vi "Generate Simulated Data.vi"(8 "error in (no error)":T5 caption="entrée d'erreur (pas d'erreur)", 11 "Type de signal":T3) -> (0 "error out":T5 caption="sortie d'erreur", 2 "Données du graphe":waveform(dbl)[](array[waveform]))   [LabVIEW 2018, in "Acquisition.lvlib"]
doc: "Génère des exemples de waveforms en fonction du type de signal dans l'entrée Configuration du matériel."
uses:
  Acquisition.lvlib
  <vilib>/Analysis/NI_AALBase.lvlib
  Signal Type.ctl
  Hardware Configuration.ctl
  Logging/Logging Configuration.ctl
  Logging/Logging.lvlib
  Settings/Settings.ctl
  Settings/Settings.lvlib
panel:
  in  "Paramètres en entrée":T1={"Configuration du matériel"={"Refnum de matériel <À remplacer>"="", "Type de signal <À remplacer>"=enum."Sine Wave"}, "Configuration de l'enregistrement"={"Chemin de base du fichier journal"=path "", "Référence de fichier TDMS"=refnum}, "Mode de longueur d'onde"={"Choix du mode"=TRUE, "Commande numérique"=0.0}, "périphérique"={"Nom du périphérique"="Dev1"}}
  in  "S5":bool[](array[boolean])=[FALSE, TRUE, FALSE, TRUE]
  in  "S4":bool[](array[boolean])=[FALSE, TRUE, FALSE, FALSE]
  in  "S6":bool[](array[boolean])=[FALSE, TRUE, TRUE, FALSE]
  in  "S7":bool[](array[boolean])=[FALSE, TRUE, TRUE, TRUE]
  in  "S13":bool[](array[boolean])=[TRUE, TRUE, FALSE, TRUE]
  in  "S12":bool[](array[boolean])=[TRUE, TRUE, FALSE, FALSE]
  in  "S11":bool[](array[boolean])=[TRUE, FALSE, TRUE, TRUE]
  in  "S10":bool[](array[boolean])=[TRUE, FALSE, TRUE, FALSE]
  in  "S9":bool[](array[boolean])=[TRUE, FALSE, FALSE, TRUE]
  in  "S8":bool[](array[boolean])=[TRUE, FALSE, FALSE, FALSE]
  in  "S3":bool[](array[boolean])=[TRUE, TRUE, FALSE, FALSE]
  in  "S2":bool[](array[boolean])=[FALSE, TRUE, FALSE, FALSE]
  in  "S1":bool[](array[boolean])=[TRUE, FALSE, FALSE, FALSE]
  in  "S0":bool[](array[boolean])=[FALSE, FALSE, FALSE, FALSE]
  in  "nom du périphérique":tag="Dev1"
  out "Graphe déroulant":dynamicdata(graph)
  # "ALLO MON GROS TAPON\n\nCOMPTE TES SWITCH A L'ENDROIT AVANT QUE JE TE CASSE TES KNEECAP"
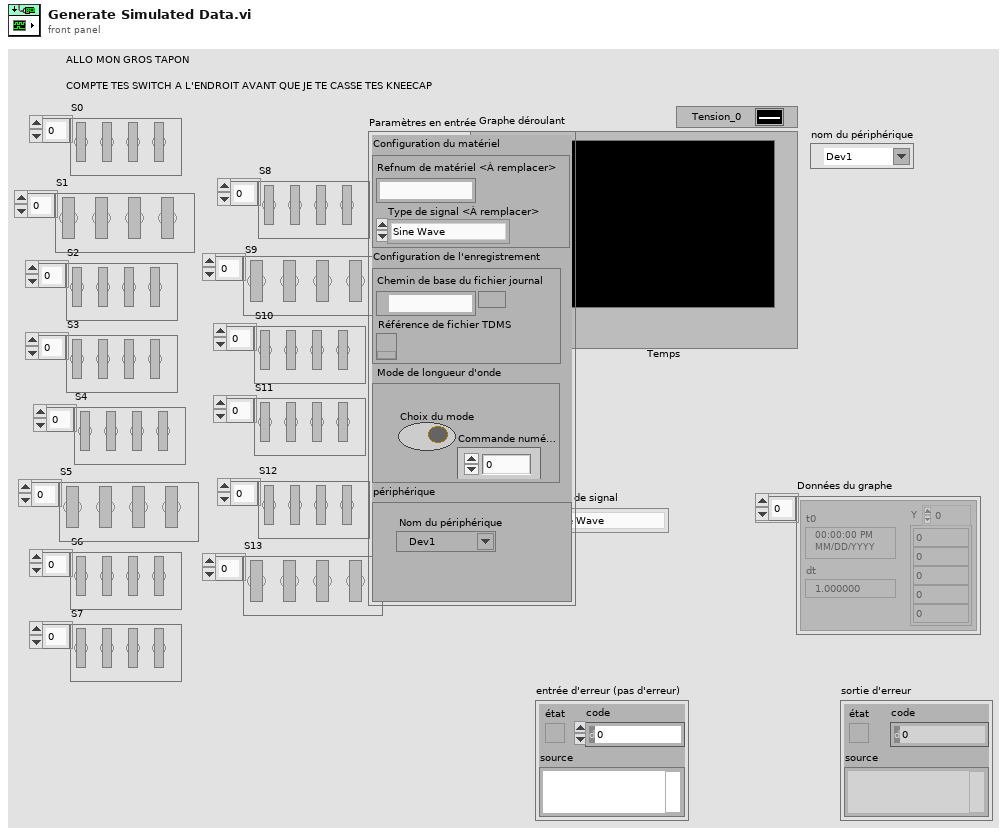
[diagram p1: front panel]
types:
  T1 = typedef "Settings.lvlib/Settings.ctl" = cluster{"Configuration du matériel":T2, "Configuration de l'enregistrement":T4, "Mode de longueur d'onde":cluster{"Choix du mode":bool, "Commande numérique":dbl}, "périphérique":cluster{"Nom du périphérique":tag}}
  T2 = typedef "Acquisition.lvlib/Hardware Configuration.ctl" = cluster{"Refnum de matériel <À remplacer>":string, "Type de signal <À remplacer>":T3}
  T3 = typedef "Acquisition.lvlib/Signal Type.ctl" = enum16{"Sine Wave", "Square with Noise", "Signal triangulaire", "Simulation DAQ"}
  T4 = typedef "Logging.lvlib/Logging Configuration.ctl" = cluster{"Chemin de base du fichier journal":path, "Référence de fichier TDMS":refnum<k34>}
  T5 = cluster{"état":bool, "code":i32, "source":string}
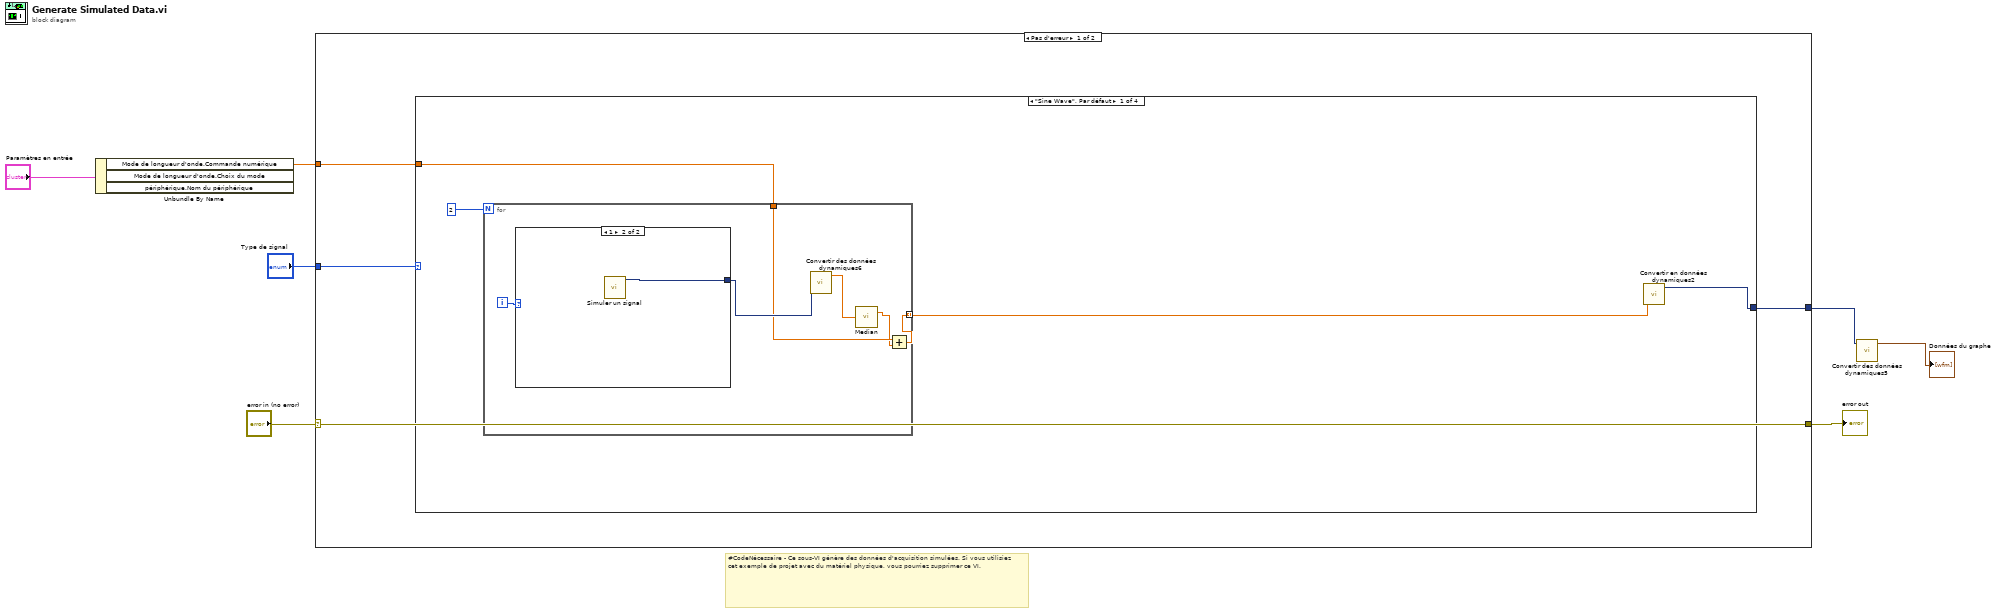
[diagram p0: block diagram]
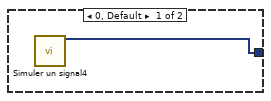
[diagram p2: hidden frame]
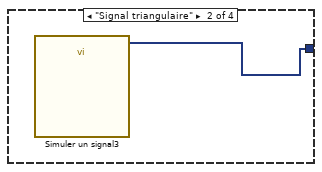
[diagram p3: hidden frame]
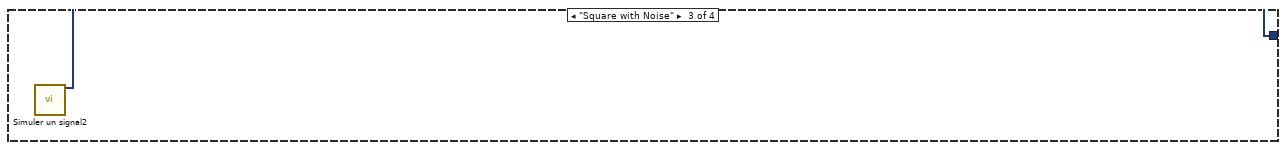
[diagram p4: hidden frame]
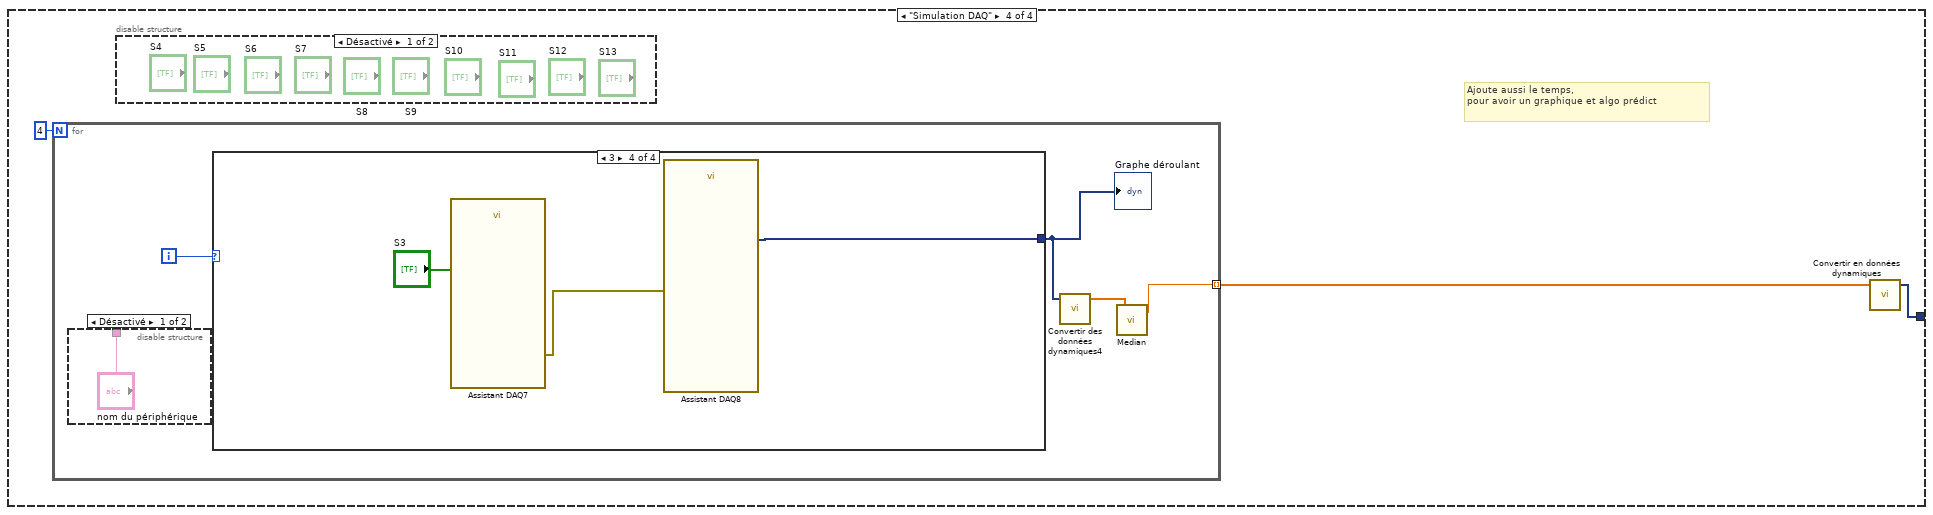
[diagram p5: hidden frame]
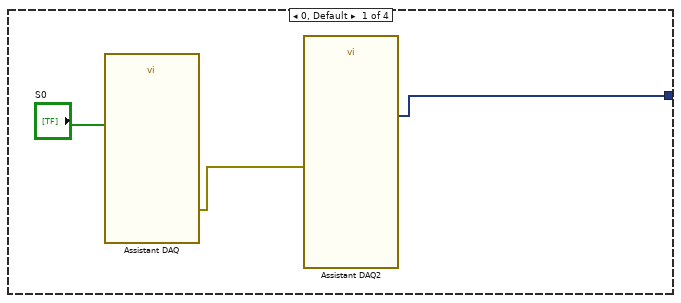
[diagram p7: hidden frame]
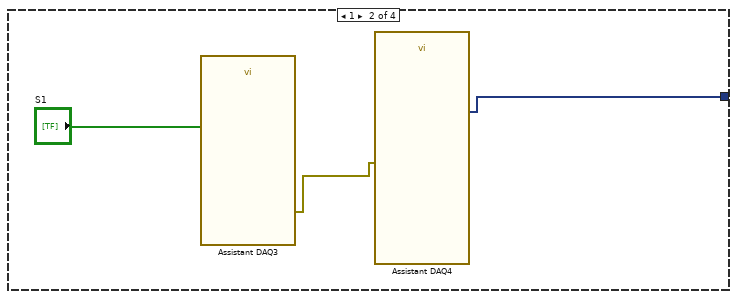
[diagram p8: hidden frame]
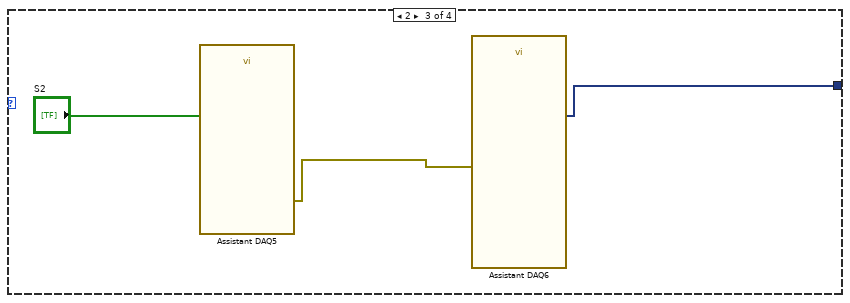
[diagram p9: hidden frame]
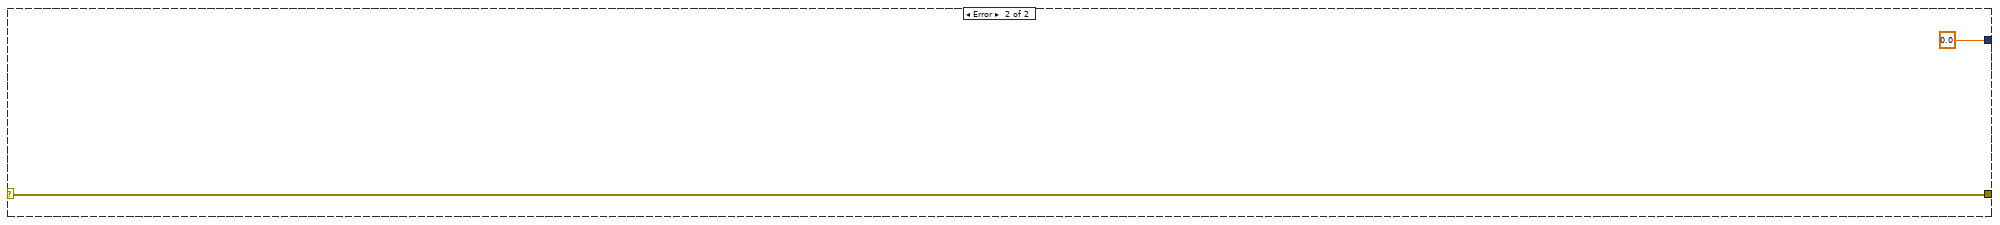
[diagram p11: hidden frame]
diagram:
  # "#CodeNécessaire - Ce sous-VI génère des données d'acquisition simulées. Si vous utilisiez cet exemple de projet avec du matériel physique, vous pourriez supprimer ce VI."
  n1 = Unbundle By Name("Paramètres en entrée") -> ("Mode de longueur d'onde.Commande numérique"=w1:dbl)  [unwired: 2 out]
  n2 = case shown="Pas d'erreur" "error in (no error)" {
    selector: "error in (no error)" -> [w11 w47]
    tunnel: [w11 w47] -> w6
    tunnel: "Type de signal" -> [w10 _]
    tunnel: [w9 0.0] -> w3
    tunnel: w1 -> [w8 _]
    frame No Error {
      n3 = case shown="\"Sine Wave\", Par défaut" w10 {
        tunnel: [w13 w24 w25 w27] -> w9
        tunnel: w8 -> [w12 _ _ _]
        frame "Sine Wave", Default {
          n4 = for {
            N: 2 -> [_]
            tunnel: [w16] -> w14 mode=indexing
            tunnel: w12 -> [w18]
            i -> [w21]
            n5 = case shown="1" w21 {
              tunnel: [w22 w23] -> w20
              frame 0, Default {
                n6 = call "Simuler un signal4"() -> ("CC"=w22:dynamicdata)  [unwired: 14 in, 1 out]
              }
              frame 1 {
                n7 = call "Simuler un signal"() -> ("Sinus avec Bruit uniforme"=w23:dynamicdata)  [unwired: 14 in, 1 out]
              }
            }
            n8 = call "Convertir des données dynamiques6"("Dynamic Data Type"=w20) -> ("Array"=w19:dbl[])  [unwired: 3 in]
            n9 = call <vilib>:"Median.vi"("X"=w19) -> ("median"=w17:dbl)  [unwired: 1 out]
            n10 = Add(x=w18, y=w17) -> (x+y=w16:dbl)
          }
          n11 = call "Convertir en données dynamiques2"("Array"=w14) -> ("Dynamic Data Type"=w13:dynamicdata)  [unwired: 3 in]
        }
        frame "Signal triangulaire" {
          n12 = call "Simuler un signal3"() -> ("Triangle"=w24:dynamicdata)  [unwired: 14 in, 1 out]
        }
        frame "Square with Noise" {
          n13 = call "Simuler un signal2"() -> ("Square with Gaussian Noise"=w25:dynamicdata)  [unwired: 14 in, 1 out]
        }
        frame "Simulation DAQ" {
          # "Ajoute aussi le temps,\npour avoir un graphique et algo prédict"
          n14 = for {
            N: 4 -> [_]
            tunnel: [w31] -> w26 mode=indexing
            i -> [w32]
            n15 = disable-structure shown="Désactivé" {
              disable-tunnel: ["nom du périphérique" _] -> _
              frame Disabled {
              }
              frame Enabled {
              }
            }
            n16 = case shown="3" w32 {
              tunnel: [w35 w37 w40 w44] -> w30
              frame 0, Default {
                n17 = call "Assistant DAQ"("data"="S0") -> ("error out"=w36:errorcluster)  [unwired: 17 in, 1 out]
                n18 = call "Assistant DAQ2"("error in"=w36) -> ("data"=w35:dynamicdata)  [unwired: 16 in, 2 out]
              }
              frame 1 {
                n19 = call "Assistant DAQ3"("data"="S1") -> ("error out"=w38:errorcluster)  [unwired: 17 in, 1 out]
                n20 = call "Assistant DAQ4"("error in"=w38) -> ("data"=w37:dynamicdata)  [unwired: 16 in, 2 out]
              }
              frame 2 {
                n21 = call "Assistant DAQ5"("data"="S2") -> ("error out"=w41:errorcluster)  [unwired: 17 in, 1 out]
                n22 = call "Assistant DAQ6"("error in"=w41) -> ("data"=w40:dynamicdata)  [unwired: 16 in, 2 out]
              }
              frame 3 {
                n23 = call "Assistant DAQ7"("data"="S3") -> ("error out"=w43:errorcluster)  [unwired: 17 in, 1 out]
                n24 = call "Assistant DAQ8"("error in"=w43) -> ("data"=w44:dynamicdata)  [unwired: 16 in, 2 out]
              }
            }
            "Graphe déroulant" <- w30
            n25 = call "Convertir des données dynamiques4"("Dynamic Data Type"=w30) -> ("Array"=w29:dbl[])  [unwired: 3 in]
            n26 = call <vilib>:"Median.vi"("X"=w29) -> ("median"=w31:dbl)  [unwired: 1 out]
          }
          n27 = disable-structure shown="Désactivé" {
            frame Disabled {
            }
            frame Enabled {
            }
          }
          n28 = call "Convertir en données dynamiques"("Array"=w26) -> ("Dynamic Data Type"=w27:dynamicdata)  [unwired: 3 in]
        }
      }
    }
    frame Error {
    }
  }
  "error out" <- w6
  n29 = call "Convertir des données dynamiques5"("Dynamic Data Type"=w3) -> ("Array of Waveform"=→"Données du graphe":waveform(dbl)[])  [unwired: 3 in]
